vi "ActionVIOnCompile.vi"(8 "error in (no error)":errorcluster, 11 "Device Item Ref in":T1 format="%.0x") -> (0 "error out":errorcluster)   [LabVIEW 2019, in "Instrument Addon System Explorer.lvlib"]
uses:
  Instrument Addon System Explorer.lvlib
  <vilib>/NI VeriStand/Custom Device API/Custom Device Item Ref.ctl
  Addon Shared/Types/Compiled Settings.ctl
  Addon Shared/Types/Command Parameters.ctl
  Addon Shared/Types/Linked Channel Cluster.ctl
  Addon Shared/Types/Command Channel Indeces.ctl
  Addon Shared/Types/Command Channel Index.ctl
  Addon Shared/Types/Response RT Configuration Cluster.ctl
  Addon Shared/Types/Response Parameters.ctl
  Addon Shared/Types/Response Wait Type.ctl
  Addon Shared/Types/Message Parameters.ctl
  Addon Shared/Types/Message Generation Type.ctl
  Addon Shared/Types/External Trigger Refs.ctl
  <vilib>/NI VeriStand/Custom Device API/Data Reference.ctl
  Types/Channel Lookup Cluster.ctl
  Types/Message Channel Lookup Cluster.ctl
  Addon Shared/Types/FG Control.ctl
  Addon Shared/SubVIs/Constants.vi
  <vilib>/NI VeriStand/Custom Device API/NI VeriStand - Get Item Property.vi
  <vilib>/NI VeriStand/Custom Device API/Get Item Property (U32).vi
  <vilib>/NI VeriStand/Custom Device API/Set Item Property (U32).vi
  <vilib>/NI VeriStand/Custom Device Tools/Custom Device Utility Library/NI VeriStand - Search for All Items by GUID.vi
  <vilib>/NI VeriStand/Custom Device API/Get Item Property (Double).vi
  <vilib>/NI VeriStand/Custom Device API/Get Item Property (Boolean).vi
  <vilib>/NI VeriStand/Custom Device API/Get Item Property (String).vi
  <vilib>/NI VeriStand/Custom Device API/Set Item Property (Double).vi
  <vilib>/NI VeriStand/Custom Device API/Set Item Property (Boolean).vi
  <vilib>/NI VeriStand/Custom Device API/Set Item Property (String).vi
  <vilib>/NI VeriStand/Custom Device Tools/Custom Device Utility Library/NI VeriStand - Get Target Ref.vi
  <vilib>/NI VeriStand/Custom Device API/NI VeriStand - Get Channel Data Reference.vi
  <vilib>/NI VeriStand/Custom Device Tools/Custom Device Utility Library/NI VeriStand - Get Item Ref by Relative Path.vi
  <vilib>/NI VeriStand/Custom Device API/Set Item Property (Variant).vi
  Addon Shared/Instrument Addon Shared.lvlib
  <vilib>/NI VeriStand/Custom Device API/Custom Device API.lvlib
  <vilib>/NI VeriStand/Custom Device Tools/Custom Device Utility Library/Custom Device Utility Library.lvlib
  <vilib>/NI/NIVS Inline Async API/_Data Access System Explorer/Data Access System Explorer.lvlib
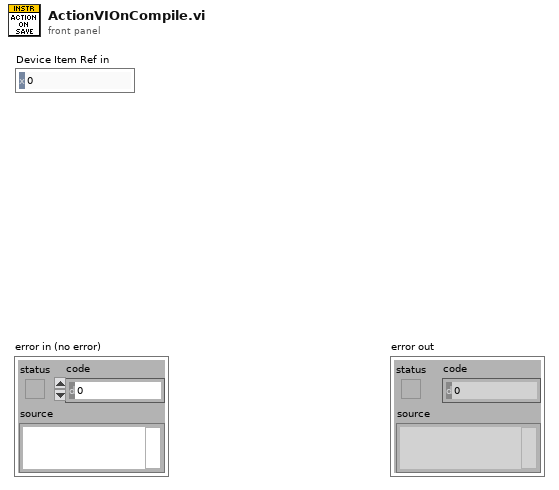
[diagram p1: front panel]
types:
  T1 = typedef "Custom Device API.lvlib/Custom Device Item Ref.ctl" = u64
  T2 = enum16{"Output/Write", "Input/Read", "Input/ReadWrite"}
  T3 = typedef "Instrument Addon Shared.lvlib/FG Control.ctl" = enum16{"Get", "Set"}
  T4 = typedef "Instrument Addon System Explorer.lvlib/Message Channel Lookup Cluster.ctl" = cluster{"Status":T1[], "Triggers":T1[], "Periodic Enable":T1[]}
  T5 = typedef "Instrument Addon Shared.lvlib/Compiled Settings.ctl" = cluster{"Command Parameters":T6[], "Command Indeces":T8[], "MetaData Lookup":variant, "Name":string, "Data Lookup":variant, "Response Parameters":T10[], "Message Generation Settings":T13[], "Wait Value Lookup":variant, "Decimation":u32, "External Channels":T15}
  T6 = typedef "Instrument Addon Shared.lvlib/Command Parameters.ctl" = cluster{"Command":string, "Linked Channels":T7[], "Pad":bool, "Length":u32, "Pad Value":u8}
  T7 = typedef "Instrument Addon Shared.lvlib/Linked Channel Cluster.ctl" = cluster{"Variable Name":string, "GUID":string}
  T8 = typedef "Instrument Addon Shared.lvlib/Command Channel Indeces.ctl" = cluster{"Channels":T9[]}
  T9 = typedef "Instrument Addon Shared.lvlib/Command Channel Index.ctl" = cluster{"Data Index":i32, "Data Length":i32}
  T10 = typedef "Instrument Addon Shared.lvlib/Response RT Configuration Cluster.ctl" = cluster{"Reponse Parameters":T11, "Use?":bool}
  T11 = typedef "Instrument Addon Shared.lvlib/Response Parameters.ctl" = cluster{"Response":string, "Linked Channels":T7[], "Type Value":dbl, "Wait Type":T12, "Use Channel":bool, "Channel Path":string}
  T12 = typedef "Instrument Addon Shared.lvlib/Response Wait Type.ctl" = enum16{"Byte Count", "Wait sec"}
  T13 = typedef "Instrument Addon Shared.lvlib/Message Parameters.ctl" = cluster{"Generation Type":T14, "Period":dbl, "Include Protection":bool, "Type":string}
  T14 = typedef "Instrument Addon Shared.lvlib/Message Generation Type.ctl" = enum16{"Trigger Only", "Periodic & Trigger", "Value Change & Trigger"}
  T15 = typedef "Instrument Addon Shared.lvlib/External Trigger Refs.ctl" = cluster{"Channels":T16[], "Triggers":T16[], "Values":dbl[]}
  T16 = typedef "Custom Device API.lvlib/Data Reference.ctl" = i32
  T17 = cluster{"Name":string, "Type":enum16{"Output/Write", "Input/Read", "Input/ReadWrite"}, "VS Refs":T1[]}
  T18 = typedef "Instrument Addon System Explorer.lvlib/Channel Lookup Cluster.ctl" = cluster{"Lookup":variant, "Index":i32, "Refs":T1[]}
  T19 = typedef "Custom Device API.lvlib/Custom Device Item Info.ctl" = cluster{"Name":string, "Is Channel":bool, "GUID":string, "Is Waveform":bool}
  T20 = typedef "Instrument Addon Shared.lvlib/Trigger Parameters.ctl" = cluster{"Use Channel":bool, "Channel Path":string}
  T21 = cluster{"Name":string, "Type":enum16{"Output/Write", "Input/Read", "Input/ReadWrite"}, "VS Refs":T1[]}[]
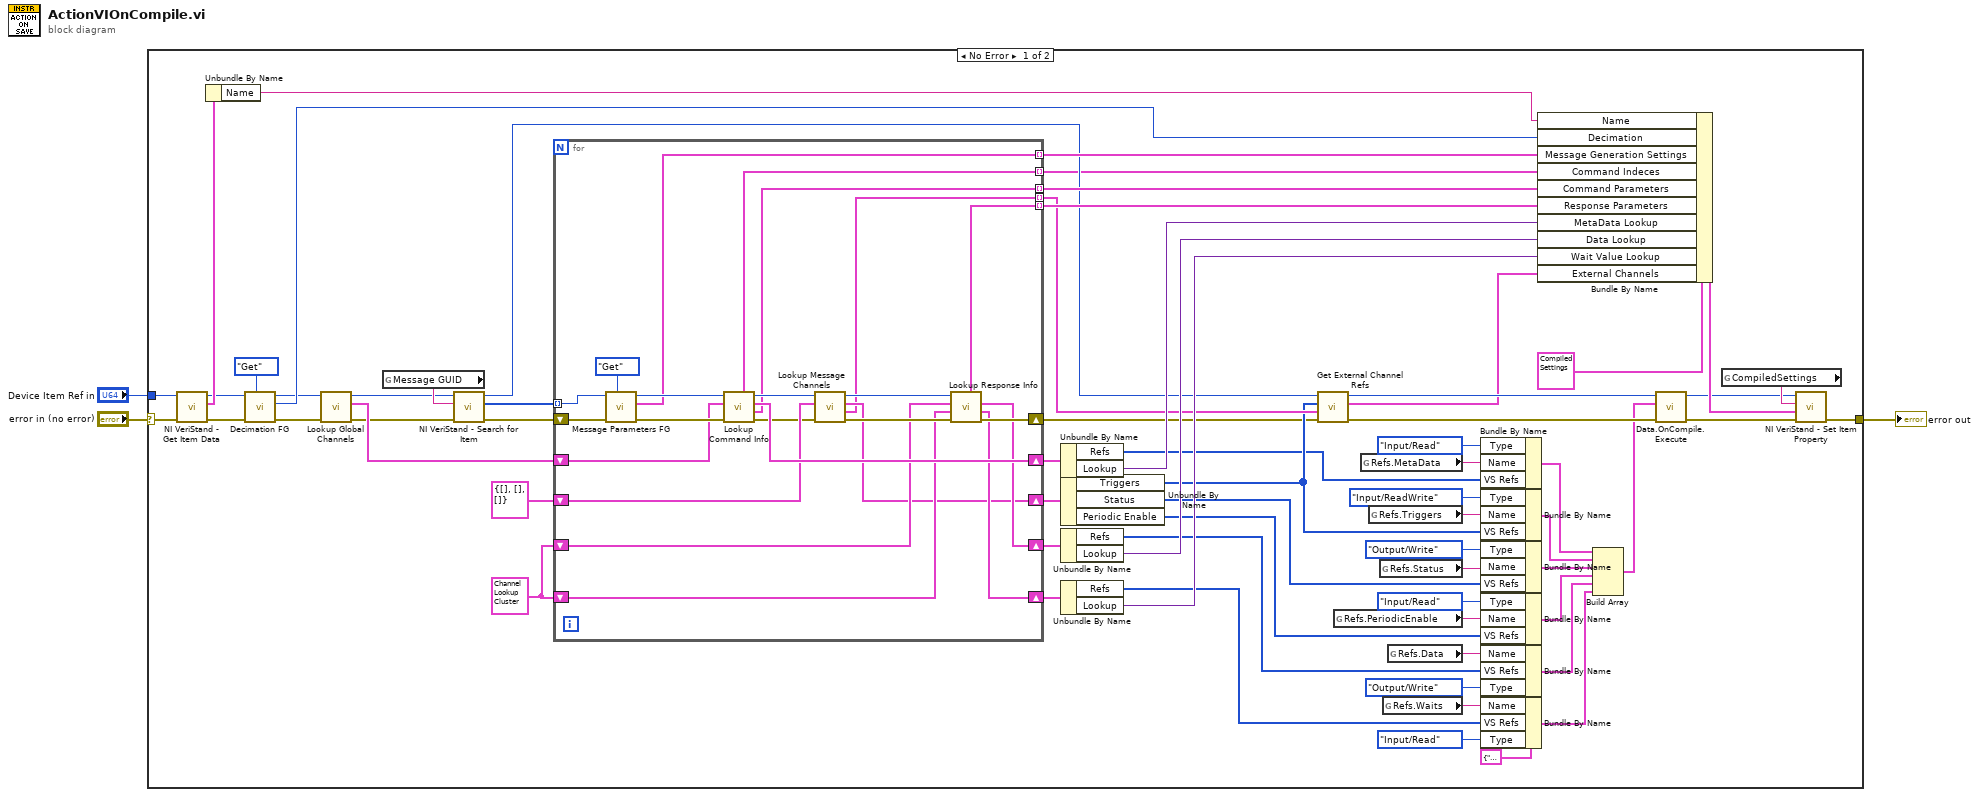
[diagram p0: block diagram]
diagram:
  n1 = case shown="No Error" "error in (no error)" {
    selector: "error in (no error)" -> [w45 w94]
    tunnel: [w44 w94] -> w2
    tunnel: "Device Item Ref in" -> [w46 _]
    frame No Error {
      w12 = T17 {"Name"="", "Type"=enum."Output/Write", "VS Refs"=[]} ("Group")
      w61 = T18 {"Lookup"=variant, "Index"=0, "Refs"=[]} ("Channel Lookup Info")
      n2 = call <vilib>:"NI VeriStand - Get Item Data.vi"("error in (no error)"=w45, "Item Ref in"=w46) -> ("error out"=w48:errorcluster, "Item Info"=w65:T19, "Item Ref out"=w49:T1)  [unwired: 6 in, 1 out]
      n3 = Unbundle By Name(w65) -> ("Name"=w10:string)
      n4 = call "Decimation FG.vi"("Action"=FG_Control."Get", "error in (no error)"=w48, "Device Item Ref in"=w49) -> ("error out"=w40:errorcluster, "Decimation out"=w51:u32, "Item Ref out"=w41:T1)  [unwired: 6 in]
      n5 = call "Lookup Global Channels.vi"("error in (no error)"=w40, "Item Ref in"=w41) -> ("error out"=w39:errorcluster, "Channel Lookup Info"=w62:T18, "Section Ref out"=w50:T1)  [unwired: 7 in]
      n6 = global read "Constants.vi" "Message GUID"() -> (w70:string)
      n7 = call-poly <vilib>:"NI VeriStand - Search for Item.vi"("error in"=w39, "Item GUID"=w70, "Section Ref in"=w50) -> ("error out"=w68:errorcluster, "Item Refs"=w69:T1[], "Section Ref out"=w31:T1)  [unwired: 5 in, 1 out]
      n8 = for {
        tunnel: w69 -> [w89] mode=indexing
        tunnel: [w75] -> w66 mode=indexing
        shift-right: [w92] -> w32
        shift-left: w68 -> [w91]
        tunnel: [w80] -> w64 mode=indexing
        tunnel: [w74] -> w63 mode=indexing
        shift-right: [w76] -> w55
        shift-left: T4 {"Status"=[], "Triggers"=[], "Periodic Enable"=[]} -> [w78]
        shift-right: [w85] -> w60
        shift-left: w62 -> [w86]
        shift-right: [w83] -> w58
        shift-left: w61 -> [w84]
        shift-right: [w82] -> w54
        shift-left: w61 -> [w81]
        tunnel: [w73] -> w47 mode=indexing
        tunnel: [w71] -> w4 mode=indexing
        n9 = call "Message Parameters FG.vi"("Action"=FG_Control."Get", "error in (no error)"=w91, "Item Ref in"=w89) -> ("error out"=w90:errorcluster, "Message Settings out"=w74:T13, "Item Ref out"=w88:T1)  [unwired: 6 in]
        n10 = call "Lookup Command Info.vi"("error in (no error)"=w90, "Channel Lookup Info in"=w86, "Item Ref in"=w88) -> ("error out"=w72:errorcluster, "Command Parameters"=w75:T6, "Channel Lookup Info out"=w85:T18, "Section Ref out"=w79:T1, "Command Channel Indeces"=w71:T8)  [unwired: 4 in]
        n11 = call "Lookup Message Channels.vi"("error in (no error)"=w72, "Message Channels in"=w78, "Section Ref in"=w79) -> ("error out"=w93:errorcluster, "Trigger Parameters"=w73:T20, "Message Channels out"=w76:T4, "Section Ref out"=w77:T1)  [unwired: 5 in]
        n12 = call "Lookup Response Info.vi"("error in (no error)"=w93, "Wait Value Channel Lookup Info"=w81, "Resp Channel Lookup Info"=w84, "Section Ref in"=w77) -> ("error out"=w92:errorcluster, "Wait Value Channel Lookup Info out"=w82:T18, "Resp Channel Lookup Info out"=w83:T18, "Response Info"=w80:T10)  [unwired: 3 in, 1 out]
      }
      n13 = Unbundle By Name(w60) -> ("Refs"=w9:T1[], "Lookup"=w59:variant)
      n14 = Unbundle By Name(w55) -> ("Triggers"=w33:T1[], "Status"=w8:T1[], "Periodic Enable"=w36:T1[])
      n15 = Unbundle By Name(w58) -> ("Refs"=w7:T1[], "Lookup"=w57:variant)
      n16 = Unbundle By Name(w54) -> ("Refs"=w6:T1[], "Lookup"=w53:variant)
      n17 = call "Get External Channel Refs.vi"("error in (no error)"=w32, "Triggers"=w47, "Internal Trigger Refs"=w33, "Device Ref in"=w31) -> ("error out"=w35:errorcluster, "Refs"=w5:T15, "Item Ref out"=w34:T1)  [unwired: 5 in]
      n18 = global read "Constants.vi" "Refs.PeriodicEnable"() -> (w28:string)
      n19 = global read "Constants.vi" "Refs.MetaData"() -> (w25:string)
      n20 = global read "Constants.vi" "Refs.Triggers"() -> (w26:string)
      n21 = global read "Constants.vi" "Refs.Status"() -> (w27:string)
      n22 = global read "Constants.vi" "Refs.Waits"() -> (w29:string)
      n23 = global read "Constants.vi" "Refs.Data"() -> (w30:string)
      n24 = Bundle By Name(cluster=w12, "Type"=T2."Input/Read", "Name"=w25, "VS Refs"=w9) -> (w18:T17)
      n25 = Bundle By Name(cluster=w12, "Type"=T2."Input/ReadWrite", "Name"=w26, "VS Refs"=w33) -> (w17:T17)
      n26 = Bundle By Name(cluster=w12, "Type"=T2."Output/Write", "Name"=w27, "VS Refs"=w8) -> (w16:T17)
      n27 = Bundle By Name(cluster=w12, "Type"=T2."Input/Read", "Name"=w28, "VS Refs"=w36) -> (w15:T17)
      n28 = Bundle By Name(cluster=w12, "Name"=w30, "VS Refs"=w7, "Type"=T2."Output/Write") -> (w14:T17)
      n29 = Bundle By Name(cluster=w12, "Name"=w29, "VS Refs"=w6, "Type"=T2."Input/Read") -> (w13:T17)
      n30 = Bundle By Name(cluster=T5 {"Command Parameters"=[], "Command Indeces"=[], "MetaData Lookup"=variant, "Name"="", "Data Lookup"=variant, "Response Parameters"=[], "Message Generation Settings"=[], "Wait Value Lookup"=variant, "Decimation"=0, "External Channels"={"Channels"=[], "Triggers"=[], "Values"=[]}} ("Parameters"), "Name"=w10, "Decimation"=w51, "Message Generation Settings"=w63, "Command Indeces"=w4, "Command Parameters"=w66, "Response Parameters"=w64, "MetaData Lookup"=w59, "Data Lookup"=w57, "Wait Value Lookup"=w53, "External Channels"=w5) -> (w43:T5)
      n31 = Build Array(w18, w17, w16, w15, w14, w13) -> (w11:T21)
      n32 = call <vilib>:"Data.OnCompile.Execute.vi"("error in"=w35, "VS Ref Groups"=w11, "Custom Device Ref"=w34) -> ("error out"=w37:errorcluster, "Custom Device Ref"=w38:T1)  [unwired: 7 in]
      n33 = global read "Constants.vi" "CompiledSettings"() -> (w42:string)
      n34 = call-poly <vilib>:"NI VeriStand - Set Item Property.vi"("error in (no error)"=w37, "Value"=w43, "Property Name"=w42, "Item Ref in"=w38) -> ("error out"=w44:errorcluster)  [unwired: 5 in, 2 out]
    }
    frame Error {
    }
  }
  "error out" <- w2
